vi "Guardar Datos espectros.vi"(10 "Data folder":path, 11 "Data Espect":T1(array[cluster])) -> ()   [LabVIEW 2012]
uses:
  <vilib>/Utility/file.llb/Write To Spreadsheet File (string).vi
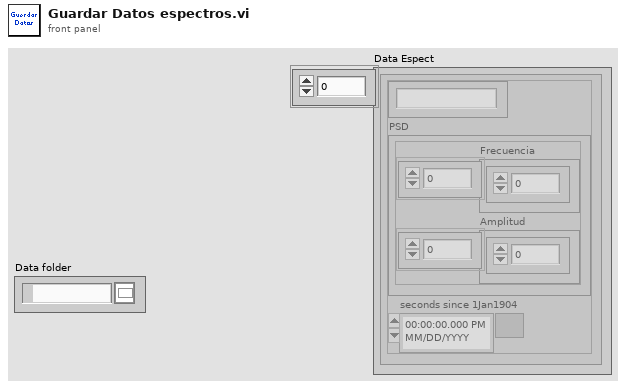
[diagram p1: front panel]
types:
  T1 = cluster{"String":string, "PSD":cluster{"Frecuencia":dbl[], "Amplitud":dbl[]}, "seconds since 1Jan1904":timestamp}[]
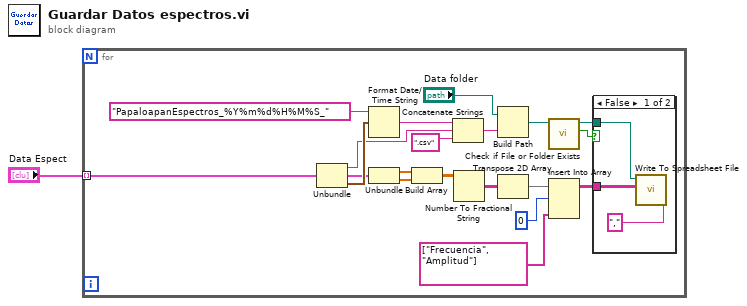
[diagram p0: block diagram]
diagram:
  n1 = for {
    tunnel: "Data Espect" -> [w21] mode=indexing
    n2 = Unbundle(w21) -> ("String"=w3:string, "PSD"=w19:cluster{"Frecuencia":dbl[], "Amplitud":dbl[]}, "seconds since 1Jan1904"=w20:timestamp)
    n3 = Format Date/Time String(time format string (%c)="PapaloapanEspectros_%Y%m%d%H%M%S_", seconds (now)=w20) -> (date/time string=w4:string)  [unwired: 1 in]
    n4 = Unbundle(w19) -> ("Frecuencia"=w18:dbl[], "Amplitud"=w17:dbl[])
    n5 = Build Array(w18, w17) -> (w16:dbl[][])
    n6 = Concatenate Strings(w4, w3, ".csv" ("string")) -> (w2:string)
    n7 = Number To Fractional String(number=w16) -> (F-format string=w7:string[][])  [unwired: 3 in]
    n8 = Build Path(base path="Data folder", name or relative path=w2) -> (appended path=w11:path)
    n9 = Transpose 2D Array(2D array=w7) -> (transposed array=w6:string[][])
    n10 = call <vilib>:"Check if File or Folder Exists.vi"("path"=w11) -> ("file or folder exists?"=w8:bool, "dup path"=w10:path)  [unwired: 8 in, 1 out]
    n11 = Insert Into Array(array=w6, index (row)=0, new element=string[] ["Frecuencia", "Amplitud"]) -> (w9:string[][])  [unwired: 1 in]
    n12 = case shown="False" w8 {
      tunnel: w10 -> [w24 _]
      tunnel: w9 -> [w23 _]
      frame False {
        n13 = call-poly <vilib>:"Write To Spreadsheet File.vi"("delimiter (\\t)"="," ("delimiter (\\t)"), "2D data"=w23, "file path (dialog if empty)"=w24) -> ()  [unwired: 5 in, 1 out]
      }
      frame True {
      }
    }
  }
